vi "ArcadeMode.vi"(9 "RightPower":dbl(slide) scale=0.0..10.0, 10 "ForwardPower":dbl(slide) scale=0.0..10.0) -> (1 "RightPower":dbl(slide) scale=0.0..10.0, 2 "LeftPower":dbl(slide) scale=0.0..10.0)   [LabVIEW 2013]
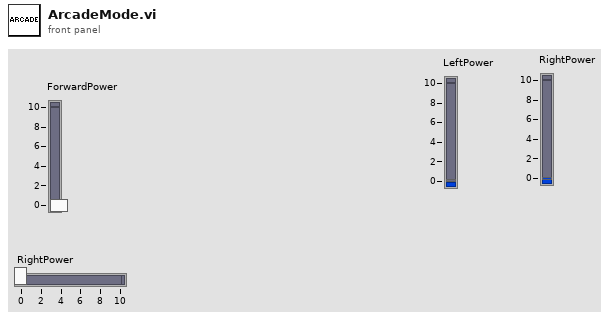
[diagram p1: front panel]
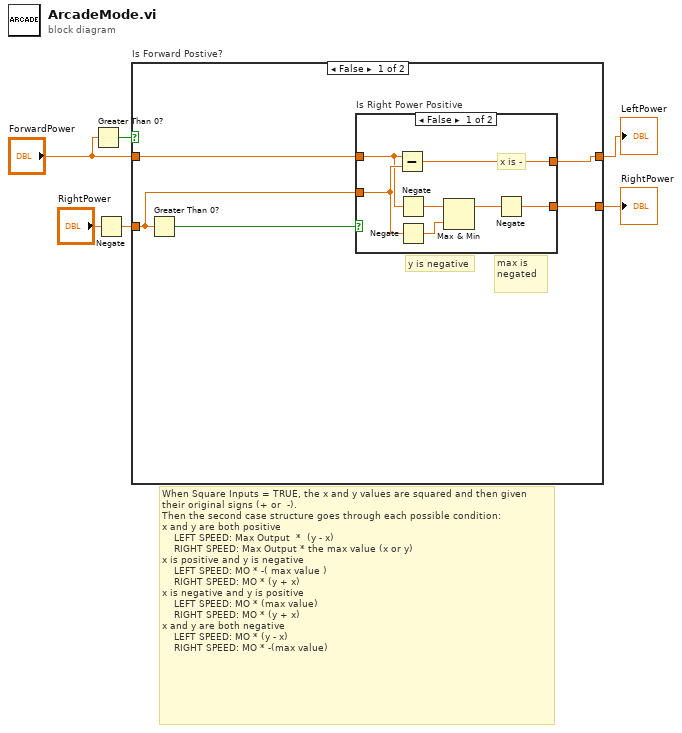
[diagram p0: block diagram]
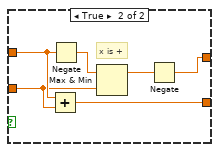
[diagram p2: hidden frame]
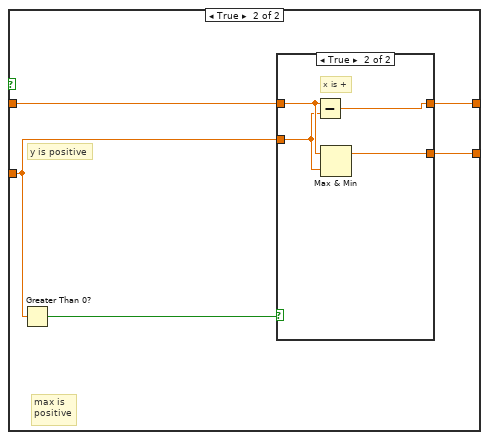
[diagram p3: hidden frame]
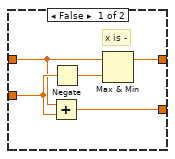
[diagram p4: hidden frame]
diagram:
  # "When Square Inputs = TRUE, the x and y values are squared and then given their original signs (+ or  -).\nThen the second case structure goes through each possible condition:\nx and y are both positive\n    LEFT SPEED: Max Output  *  (y - x)\n    RIGHT SPEED: Max Output * the max value (x or y)\nx is positive and y is negative\n    LEFT SPEED: MO * -( max value )\n    RIGHT SPEED: MO * (y + x)\nx is negative and y is positive\n    LEFT SPEED: MO * (max value)\n    RIGHT SPEED: MO * (y + x) \nx and y are both negative\n    LEFT SPEED: MO * (y - x)\n    RIGHT SPEED: MO * -(max value)"
  n1 = Greater Than 0?(x="ForwardPower") -> (x > 0?=w6:bool)
  n2 = Negate(x="RightPower") -> (-x=w1:dbl)
  n3 = case "Is Forward Postive?" shown="False" w6 {
    tunnel: w1 -> [w10 w28]
    tunnel: "ForwardPower" -> [w9 w27]
    tunnel: [w8 w26] -> w3
    tunnel: [w7 w25] -> w2
    frame False {
      # "max is negated"
      # "y is negative"
      n4 = Greater Than 0?(x=w10) -> (x > 0?=w11:bool)
      n5 = case "Is Right Power Positive" shown="False" w11 {
        tunnel: w10 -> [w18 w20]
        tunnel: w9 -> [w16 w21]
        tunnel: [w12 w22] -> w8
        tunnel: [w13 w19] -> w7
        frame False {
          # "x is -"
          n6 = Subtract(x=w16, y=w18) -> (x-y=w12:dbl)
          n7 = Negate(x=w16) -> (-x=w17:dbl)
          n8 = Negate(x=w18) -> (-x=w15:dbl)
          n9 = Max & Min(x=w17, y=w15) -> (max(x,y)=w14:dbl)  [unwired: 1 out]
          n10 = Negate(x=w14) -> (-x=w13:dbl)
        }
        frame True {
          # "x is +"
          n11 = Add(x=w21, y=w20) -> (x+y=w19:dbl)
          n12 = Negate(x=w21) -> (-x=w24:dbl)
          n13 = Max & Min(x=w24, y=w20) -> (max(x,y)=w23:dbl)  [unwired: 1 out]
          n14 = Negate(x=w23) -> (-x=w22:dbl)
        }
      }
    }
    frame True {
      # "max is\npositive"
      # "y is positive"
      n15 = Greater Than 0?(x=w28) -> (x > 0?=w29:bool)
      n16 = case shown="True" w29 {
        tunnel: w28 -> [w34 w36]
        tunnel: w27 -> [w31 w37]
        tunnel: [w32 w35] -> w26
        tunnel: [w30 w38] -> w25
        frame False {
          # "x is -"
          n17 = Add(x=w31, y=w34) -> (x+y=w30:dbl)
          n18 = Negate(x=w34) -> (-x=w33:dbl)
          n19 = Max & Min(x=w31, y=w33) -> (max(x,y)=w32:dbl)  [unwired: 1 out]
        }
        frame True {
          # "x is +"
          n20 = Subtract(x=w37, y=w36) -> (x-y=w35:dbl)
          n21 = Max & Min(x=w37, y=w36) -> (max(x,y)=w38:dbl)  [unwired: 1 out]
        }
      }
    }
  }
  "LeftPower" <- w3
  "RightPower" <- w2
